vi "_GetPeakProperties.vi"(4 "Peak":T1, 5 "Intensities":dbl[](array[numeric]), 6 "Masses":dbl[](array[numeric]), 7 "Location":dbl) -> (0 "Baseline":dbl, 1 "FWHM":dbl, 2 "Height":dbl, 3 "Mass":dbl)   [LabVIEW 2015]
uses:
  Type/_Peak Property.ctl
panel:
  out "HalfHeight":dbl
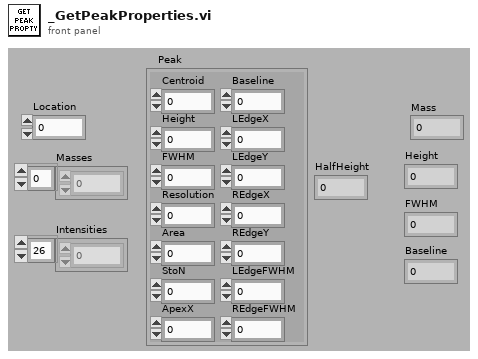
[diagram p1: front panel]
types:
  T1 = typedef "_Peak Property.ctl" = cluster{"Centroid":dbl, "Height":dbl, "FWHM":dbl, "Resolution":dbl, "Area":dbl, "StoN":dbl, "ApexX":dbl, "Baseline":dbl, "LEdgeX":dbl, "LEdgeY":dbl, "REdgeX":dbl, "REdgeY":dbl, "LEdgeFWHM":dbl, "REdgeFWHM":dbl}
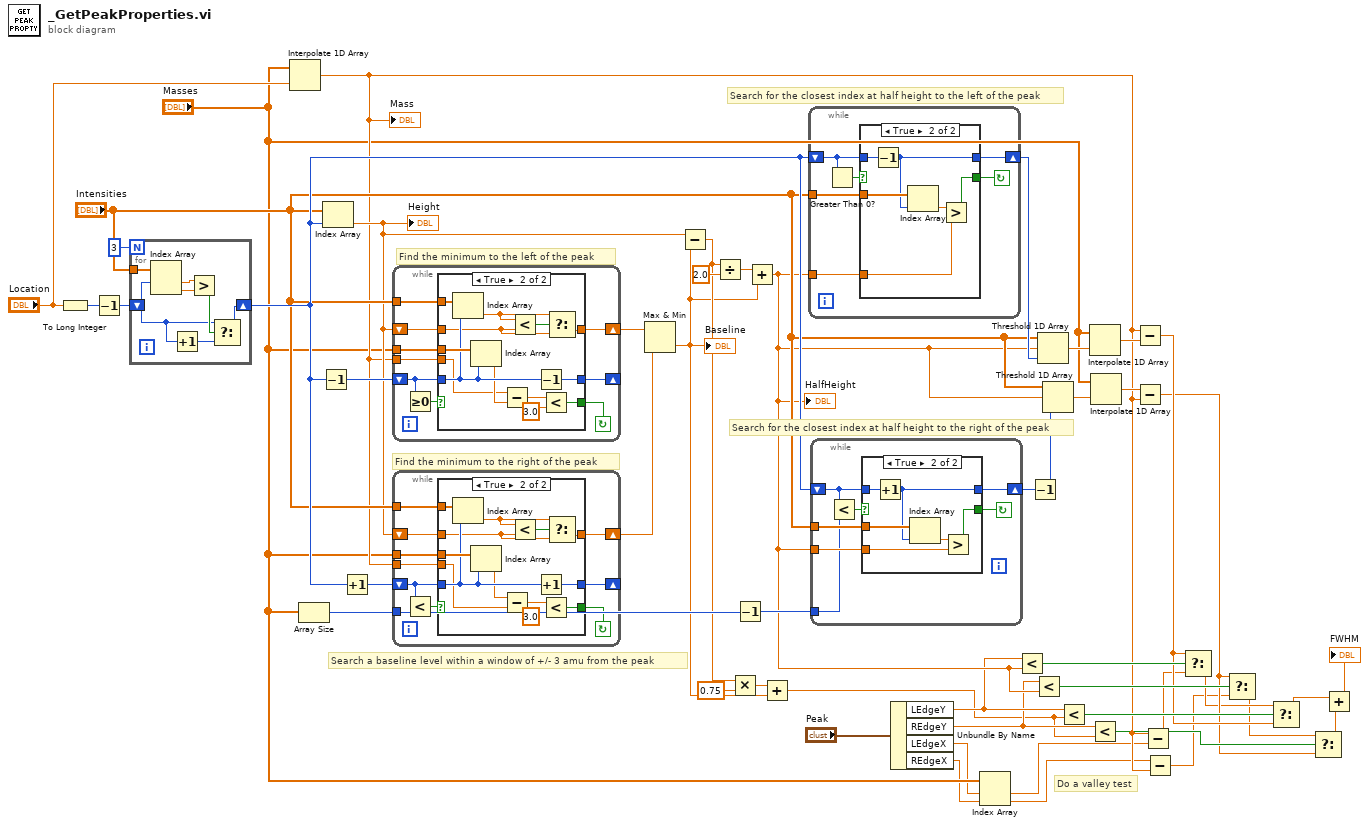
[diagram p0: block diagram]
diagram:
  # "Do a valley test"
  # "Search for the closest index at half height to the right of the peak"
  # "Search for the closest index at half height to the left of the peak"
  # "Search a baseline level within a window of +/- 3 amu from the peak"
  # "Find the minimum to the right of the peak"
  # "Find the minimum to the left of the peak"
  n1 = To Long Integer(number="Location") -> (32bit integer=w31:i32)
  n2 = Decrement(x=w31) -> (x-1=w42:i32)
  n3 = for {
    N: 3 -> [_]
    shift-right: [w54] -> w39
    shift-left: w42 -> [w51]
    tunnel: "Intensities" -> [w57]
    n4 = Index Array(array=w57, index #1=w51) -> (element #1=w55:dbl, element #2=w56:dbl)  [unwired: 1 in]
    n5 = Increment(x=w51) -> (x+1=w52:i32)
    n6 = Greater?(x=w55, y=w56) -> (0:w53:bool)
    n7 = Select(t=w51, s=w53, f=w52) -> (s? t:f=w54:i32)
  }
  n8 = Interpolate 1D Array(1:"Location", 2:"Masses") -> (0:w8:dbl)
  "Mass" <- w8
  n9 = Array Size(array="Masses") -> (size(s)=w38:i32)
  n10 = Decrement(x=w39) -> (x-1=w50:i32)
  n11 = Index Array(array="Intensities", index=w39) -> (element=w29:dbl)
  "Height" <- w29
  n12 = Increment(x=w39) -> (x+1=w49:i32)
  n13 = while {
    shift-right: [w61] -> w48
    shift-left: w29 -> [w62]
    shift-right: [w66] -> _
    shift-left: w50 -> [w65]
    tunnel: w8 -> [w60]
    tunnel: "Masses" -> [w59]
    tunnel: "Intensities" -> [w58]
    stop <- w63 continue-if-true
    n14 = Greater Or Equal To 0?(x=w65) -> (x >= 0?=w64:bool)
    n15 = case shown="True" w64 {
      selector: w64 -> [w69 _]
      tunnel: [w68 w82] -> w66
      tunnel: w65 -> [w68 w79]
      tunnel: [w69 w70] -> w63
      tunnel: [w67 w76] -> w61
      tunnel: w62 -> [w67 w75]
      tunnel: w60 -> [_ w73]
      tunnel: w59 -> [_ w81]
      tunnel: w58 -> [_ w80]
      frame False {
      }
      frame True {
        n16 = Index Array(array=w80, index=w79) -> (element=w77:dbl)
        n17 = Index Array(array=w81, index=w79) -> (element=w74:dbl)
        n18 = Subtract(x=w73, y=w74) -> (x-y=w72:dbl)
        n19 = Less?(x=w77, y=w75) -> (x < y?=w78:bool)
        n20 = Decrement(x=w79) -> (x-1=w82:i32)
        n21 = Less?(x=w72, y=3.0) -> (x < y?=w70:bool)
        n22 = Select(t=w77, s=w78, f=w75) -> (s? t:f=w76:dbl)
      }
    }
  }
  n23 = while {
    shift-right: [w88] -> w47
    shift-left: w29 -> [w89]
    shift-right: [w92] -> _
    shift-left: w49 -> [w84]
    tunnel: w8 -> [w87]
    tunnel: "Masses" -> [w86]
    tunnel: "Intensities" -> [w85]
    tunnel: w38 -> [w83]
    stop <- w90 continue-if-true
    n24 = Less?(x=w84, y=w83) -> (x < y?=w91:bool)
    n25 = case shown="True" w91 {
      selector: w91 -> [w95 _]
      tunnel: [w94 w108] -> w92
      tunnel: w84 -> [w94 w105]
      tunnel: [w95 w98] -> w90
      tunnel: [w93 w102] -> w88
      tunnel: w89 -> [w93 w101]
      tunnel: w87 -> [_ w96]
      tunnel: w86 -> [_ w107]
      tunnel: w85 -> [_ w106]
      frame False {
      }
      frame True {
        n26 = Index Array(array=w106, index=w105) -> (element=w103:dbl)
        n27 = Index Array(array=w107, index=w105) -> (element=w97:dbl)
        n28 = Subtract(x=w97, y=w96) -> (x-y=w100:dbl)
        n29 = Less?(x=w103, y=w101) -> (x < y?=w104:bool)
        n30 = Increment(x=w105) -> (x+1=w108:i32)
        n31 = Less?(x=w100, y=3.0) -> (x < y?=w98:bool)
        n32 = Select(t=w103, s=w104, f=w101) -> (s? t:f=w102:dbl)
      }
    }
  }
  n33 = Max & Min(x=w48, y=w47) -> (min(x,y)=w24:dbl)  [unwired: 1 out]
  "Baseline" <- w24
  n34 = Subtract(x=w29, y=w24) -> (x-y=w27:dbl)
  n35 = Divide(x=w27, y=2.0) -> (x/y=w45:dbl)
  n36 = Multiply(x=w27, y=0.75) -> (x*y=w25:dbl)
  n37 = Decrement(x=w38) -> (x-1=w37:i32)
  n38 = Add(x=w45, y=w24) -> (x+y=w21:dbl)
  "HalfHeight" <- w21
  n39 = Add(x=w25, y=w24) -> (x+y=w9:dbl)
  n40 = while {
    tunnel: w21 -> [w109]
    shift-right: [w112] -> w44
    shift-left: w39 -> [w113]
    tunnel: "Intensities" -> [w110]
    stop <- w111 continue-if-true
    n41 = Greater Than 0?(x=w113) -> (x > 0?=w114:bool)
    n42 = case shown="True" w114 {
      selector: w114 -> [w115 _]
      tunnel: [w116 w117] -> w112
      tunnel: w113 -> [w116 w118]
      tunnel: [w115 w119] -> w111
      tunnel: w110 -> [_ w122]
      tunnel: w109 -> [_ w120]
      frame False {
      }
      frame True {
        n43 = Decrement(x=w118) -> (x-1=w117:i32)
        n44 = Index Array(array=w122, index=w117) -> (element=w121:dbl)
        n45 = Greater?(x=w121, y=w120) -> (0:w119:bool)
      }
    }
  }
  n46 = while {
    tunnel: w21 -> [w125]
    shift-right: [w128] -> w36
    shift-left: w39 -> [w123]
    tunnel: "Intensities" -> [w126]
    tunnel: w37 -> [w124]
    stop <- w127 continue-if-true
    n47 = Less?(x=w123, y=w124) -> (x < y?=w129:bool)
    n48 = case shown="True" w129 {
      selector: w129 -> [w130 _]
      tunnel: [w131 w132] -> w128
      tunnel: w123 -> [w131 w133]
      tunnel: [w130 w134] -> w127
      tunnel: w126 -> [_ w137]
      tunnel: w125 -> [_ w135]
      frame False {
      }
      frame True {
        n49 = Increment(x=w133) -> (x+1=w132:i32)
        n50 = Index Array(array=w137, index=w132) -> (element=w136:dbl)
        n51 = Greater?(x=w136, y=w135) -> (0:w134:bool)
      }
    }
  }
  n52 = Unbundle By Name("Peak") -> ("LEdgeY"=w11:dbl, "REdgeY"=w10:dbl, "LEdgeX"=w4:dbl, "REdgeX"=w2:dbl)
  n53 = Index Array(array="Masses", index #1=w4, index #2=w2) -> (element #1=w3:dbl, element #2=w1:dbl)
  n54 = Less?(x=w11, y=w21) -> (x < y?=w20:bool)
  n55 = Decrement(x=w36) -> (x-1=w35:i32)
  n56 = Less?(x=w10, y=w21) -> (x < y?=w19:bool)
  n57 = Threshold 1D Array(1:w44, 2:w21, 3:"Intensities") -> (0:w43:dbl)
  n58 = Threshold 1D Array(1:w35, 2:w21, 3:"Intensities") -> (0:w33:dbl)
  n59 = Less?(x=w11, y=w9) -> (x < y?=w23:bool)
  n60 = Interpolate 1D Array(1:w43, 2:"Masses") -> (0:w40:dbl)
  n61 = Less?(x=w10, y=w9) -> (x < y?=w22:bool)
  n62 = Interpolate 1D Array(1:w33, 2:"Masses") -> (0:w32:dbl)
  n63 = Subtract(x=w8, y=w40) -> (x-y=w18:dbl)
  n64 = Subtract(x=w32, y=w8) -> (x-y=w17:dbl)
  n65 = Subtract(x=w8, y=w3) -> (x-y=w7:dbl)
  n66 = Subtract(x=w1, y=w8) -> (x-y=w6:dbl)
  n67 = Select(t=w18, s=w20, f=w7) -> (s? t:f=w16:dbl)
  n68 = Select(t=w17, s=w19, f=w6) -> (s? t:f=w15:dbl)
  n69 = Select(t=w16, s=w23, f=w18) -> (s? t:f=w13:dbl)
  n70 = Select(t=w15, s=w22, f=w17) -> (s? t:f=w14:dbl)
  n71 = Add(x=w13, y=w14) -> (x+y=→"FWHM":dbl)
